vi "TIFF Add Image (replace).vi"(8 "error in (no error)":errorcluster, 10 "IFD Array":refnum<class "IFD.lvclass">[](array[class]), 11 "TIFF in":refnum<class "TIFF.lvclass">) -> (0 "error out":errorcluster, 3 "TIFF out":refnum<class "TIFF.lvclass">)   [LabVIEW 2016, in "TIFF.lvclass"]
uses:
  TIFF.lvclass
  IFD/IFD.lvclass
  TIFF.lvclass/TIFF.ctl
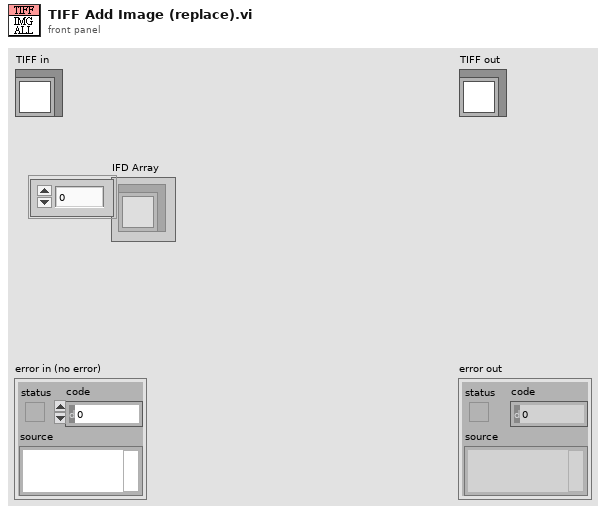
[diagram p1: front panel]
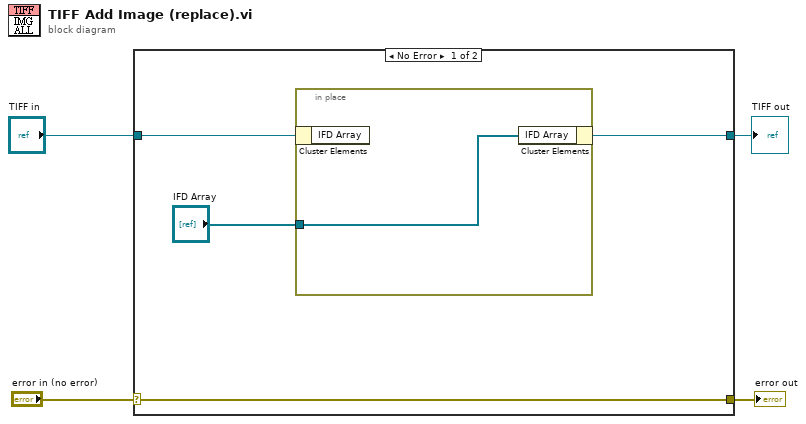
[diagram p0: block diagram]
diagram:
  n1 = case shown="No Error" "error in (no error)" {
    selector: "error in (no error)" -> [w8 w11]
    tunnel: [w8 w11] -> w3
    tunnel: [w6 w10] -> w1
    tunnel: "TIFF in" -> [w7 w10]
    frame No Error {
      n2 = in-place {
        in-place-border: "IFD Array" -> [w9]
        n3 = in-place-cluster #1(w7) -> ()  [unwired: 1 out]
        n4 = in-place-cluster #1("IFD Array"=w9) -> (w6:refnum<class "TIFF.lvclass">)
      }
    }
    frame Error {
    }
  }
  "error out" <- w3
  "TIFF out" <- w1
